vi "MV3D RGBD Get Upgrade Process.vi"(10 "pProcess":u32, 11 "handle":u32) -> (1 "function return":i32, 2 "pProcess out":u32, 3 "handle out":u32)   [LabVIEW 2015, in "Mv3dRgbd.lvlib"]
doc: "MV3D_RGBD_API MV3D_RGBD_STATUS MV3D_RGBD_GetUpgradeProcess(HANDLE handle, uint32_t* pProcess);"
uses:
  <userlib>/Mv3dRgbd/Mv3dRgbd.lvlib
  <userlib>/Mv3dRgbd/Mv3dRgbd.dll
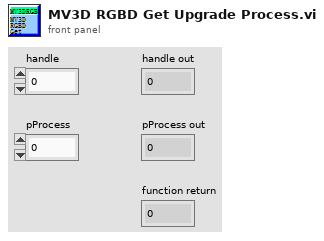
[diagram p1: front panel]
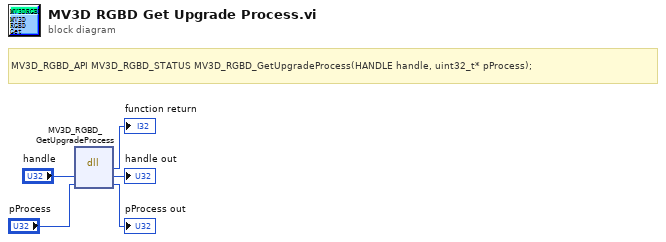
[diagram p0: block diagram]
diagram:
  # "MV3D_RGBD_API MV3D_RGBD_STATUS MV3D_RGBD_GetUpgradeProcess(HANDLE handle, uint32_t* pProcess);"
  n1 = dll-call lib="C:/Program Files (x86)/National Instruments/LabVIEW 2015/user.lib/Mv3dRgbd/Mv3dRgbd.*" fn="MV3D_RGBD_GetUpgradeProcess"("handle"="handle", "pProcess"="pProcess") -> (→"function return":i32, "handle"=→"handle out":u32, "pProcess"=→"pProcess out":u32)  [unwired: 3 in, 2 out]
